vi "writeDigital.vi"() -> ()   [LabVIEW 2017]
panel:
  out "return type":i32
  out "error out":errorcluster
  out "path out":path
  in  "error in (no error)":errorcluster
  in  "path in":path
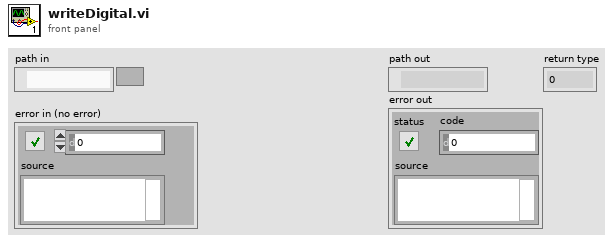
[diagram p1: front panel]
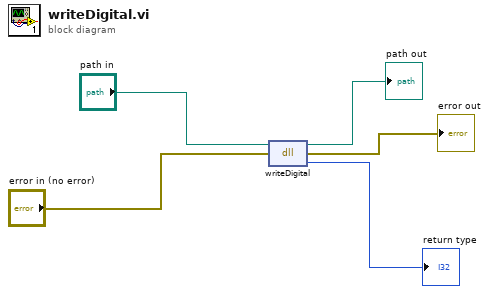
[diagram p0: block diagram]
diagram:
  n1 = dll-call lib="C:/Users/user/Documents/AyushWork/projects/writeDigital/WriteDigital/Debug/writeDigital.dll" fn="writeDigital"(path in="path in", error in="error in (no error)") -> (path out=→"path out":path, error out=→"error out":errorcluster, "return type"=→"return type":i32)  [unwired: 1 in]
